vi "TargetHit.vi"(6 "Position":T1, 8 "error in (no error)":errorcluster, 9 "Pitch":sgl, 10 "Yaw":sgl, 11 "Level in":refnum<class "Level.lvclass">) -> (0 "error out":errorcluster, 2 "Hit Targets":string[](array[string]), 3 "Level out":refnum<class "Level.lvclass">)   [LabVIEW 2015, in "Level.lvclass"]
uses:
  Level.lvclass
  3D Point.ctl
  Level.lvclass/Level.ctl
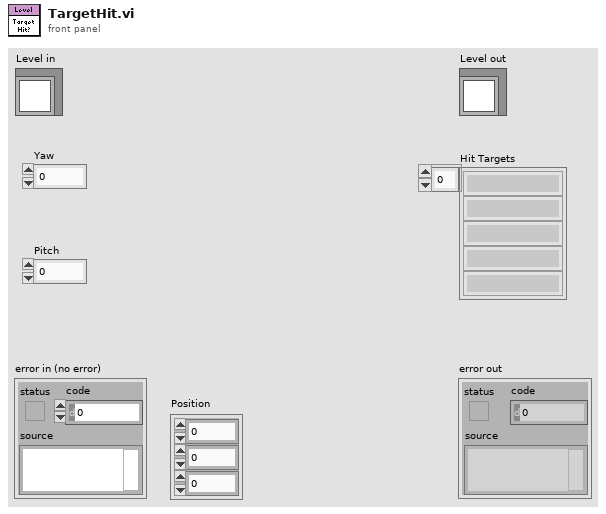
[diagram p1: front panel]
types:
  T1 = typedef "3D Point.ctl" = cluster{"X":sgl, "Y":sgl, "Z":sgl}
  T2 = cluster{"Point 1":cluster{"Z":dbl, "X":dbl}, "Point 2":cluster{"Z":dbl, "X":dbl}}
  T3 = typedef "Level.lvclass/Segment.ctl" = cluster{"Point 1":T4, "Point 2":T4}
  T4 = typedef "Level.lvclass/Point.ctl" = cluster{"Z":dbl, "X":dbl}
  T5 = cluster{"Segment":T3, "Position":T1, "Radius":sgl}[]
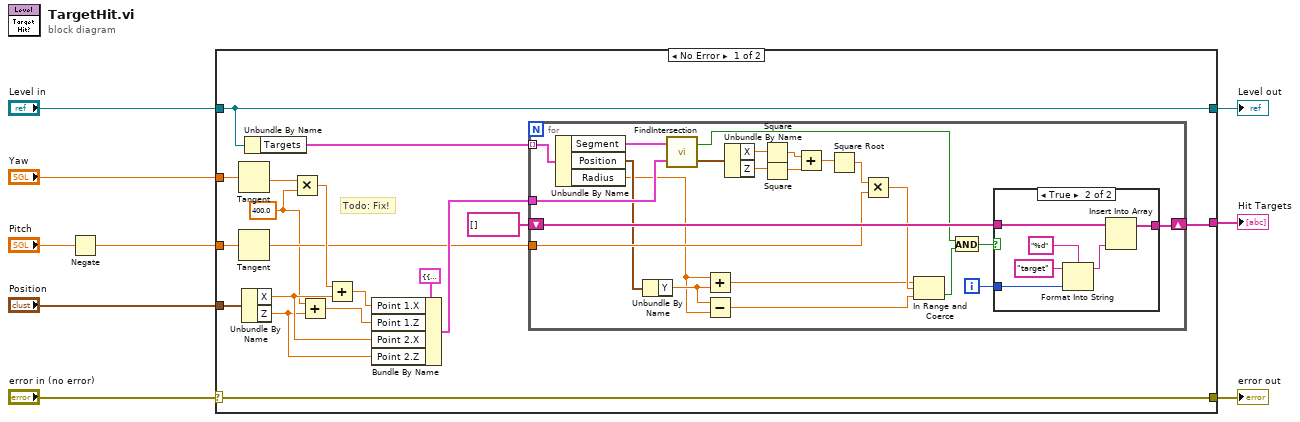
[diagram p0: block diagram]
diagram:
  n1 = Negate(x="Pitch") -> (-x=w2:sgl)
  n2 = case shown="No Error" "error in (no error)" {
    selector: "error in (no error)" -> [w27 w59]
    tunnel: [w27 w59] -> w8
    tunnel: [w26 w58] -> w6
    tunnel: "Level in" -> [w26 w58]
    tunnel: "Position" -> [w23 _]
    tunnel: [w14 _] -> w4
    tunnel: w2 -> [w12 _]
    tunnel: "Yaw" -> [w10 _]
    frame No Error {
      w11 = sgl 400.0 ("y")
      # "Todo: Fix!"
      n3 = Tangent(1:w10) -> (0:w24:sgl)
      n4 = Tangent(1:w12) -> (0:w13:sgl)
      n5 = Unbundle By Name(w23) -> ("X"=w18:sgl, "Z"=w17:sgl)
      n6 = Unbundle By Name(w26) -> ("Targets"=w25:T5)
      n7 = Multiply(x=w24, y=w11) -> (x*y=w22:sgl)
      n8 = Add(x=w11, y=w17) -> (x+y=w19:sgl)
      n9 = Add(x=w22, y=w18) -> (x+y=w20:sgl)
      n10 = Bundle By Name(cluster=T2 {"Point 1"={"Z"=0.0, "X"=0.0}, "Point 2"={"Z"=0.0, "X"=0.0}} ("Segment B"), "Point 1.X"=w20, "Point 1.Z"=w19, "Point 2.X"=w18, "Point 2.Z"=w17) -> (w16:T2)
      n11 = for {
        tunnel: w25 -> [w38] mode=indexing
        tunnel: w16 -> [w50]
        shift-right: [w48] -> w14
        shift-left: string[] [] -> [w47]
        tunnel: w13 -> [w39]
        i -> [w49]
        n12 = Unbundle By Name(w38) -> ("Segment"=w37:T3, "Position"=w36:T1, "Radius"=w34:sgl)
        n13 = Unbundle By Name(w36) -> ("Y"=w35:sgl)
        n14 = call "FindIntersection.vi"("Segment B"=w50, "Segment A"=w37) -> ("Intersection Point"=w46:cluster{"X":sgl, "Z":sgl}, "Segments Intersect?"=w29:bool)
        n15 = Add(x=w34, y=w35) -> (x+y=w32:sgl)
        n16 = Subtract(x=w35, y=w34) -> (x-y=w31:sgl)
        n17 = Unbundle By Name(w46) -> ("X"=w45:sgl, "Z"=w44:sgl)
        n18 = Square(x=w45) -> (x^2=w42:sgl)
        n19 = Square(x=w44) -> (x^2=w43:sgl)
        n20 = Add(x=w42, y=w43) -> (x+y=w41:sgl)
        n21 = Square Root(x=w41) -> (sqrt(x)=w40:sgl)
        n22 = Multiply(x=w40, y=w39) -> (x*y=w33:sgl)
        n23 = In Range and Coerce(upper limit=w32, x=w33, lower limit=w31) -> (In Range?=w30:bool)  [unwired: 1 out]
        n24 = And(x=w29, y=w30) -> (x .and. y?=w28:bool)
        n25 = case shown="True" w28 {
          tunnel: w49 -> [_ w56]
          tunnel: [w51 w53] -> w48
          tunnel: w47 -> [w51 w52]
          frame False {
          }
          frame True {
            n26 = Format Into String(format string="%d", initial string="target", w56) -> (resulting string=w54:string)  [unwired: 1 in, 1 out]
            n27 = Insert Into Array(array=w52, new element=w54) -> (w53:string[])  [unwired: 1 in]
          }
        }
      }
    }
    frame Error {
    }
  }
  "error out" <- w8
  "Level out" <- w6
  "Hit Targets" <- w4
